vi "Update.vi"(8 "error in (no error)":errorcluster, 9 "Process Variable":dbl, 10 "Setpoint":dbl, 11 "PID in":refnum<class "PID.lvclass">) -> (0 "error out":errorcluster, 3 "PID out":refnum<class "PID.lvclass">)   [LabVIEW 2024, in "PID.lvlib" / "PID.lvclass"]
uses:
  PID.lvclass
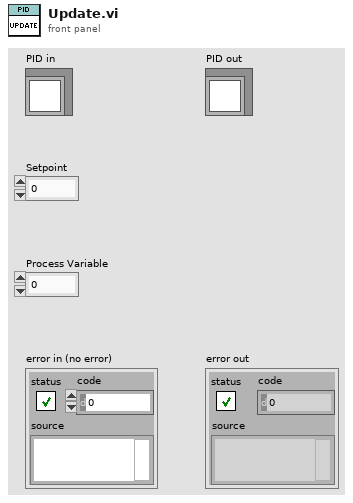
[diagram p1: front panel]
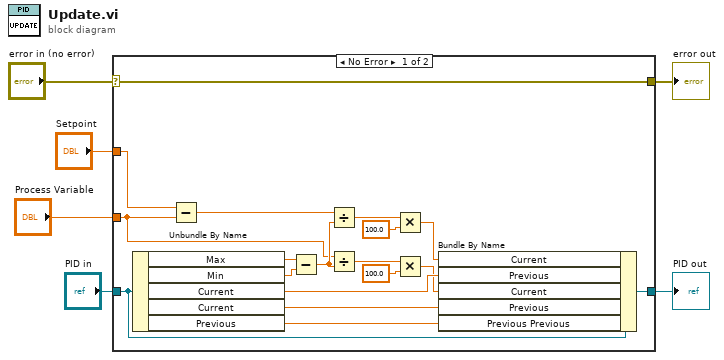
[diagram p0: block diagram]
diagram:
  n1 = case shown="No Error" "error in (no error)" {
    selector: "error in (no error)" -> [w24 w26]
    tunnel: [w24 w26] -> w5
    tunnel: [w14 w25] -> w3
    tunnel: "PID in" -> [w23 w25]
    tunnel: "Setpoint" -> [w22 _]
    tunnel: "Process Variable" -> [w10 _]
    frame No Error {
      n2 = Unbundle By Name(w23) -> ("Max"=w20:dbl, "Min"=w19:dbl, "Current"=w15:dbl, "Current"=w13:dbl, "Previous"=w12:dbl)
      n3 = Subtract(x=w22, y=w10) -> (x-y=w21:dbl)
      n4 = Subtract(x=w20, y=w19) -> (x-y=w11:dbl)
      n5 = Divide(x=w21, y=w11) -> (x/y=w18:dbl)
      n6 = Divide(x=w10, y=w11) -> (x/y=w9:dbl)
      n7 = Multiply(x=w18, y=100.0) -> (x*y=w16:dbl)
      n8 = Multiply(x=w9, y=100.0) -> (x*y=w7:dbl)
      n9 = Bundle By Name(cluster=w23, "Current"=w16, "Previous"=w15, "Current"=w7, "Previous"=w13, "Previous Previous"=w12) -> (w14:refnum<class "PID.lvclass">)
    }
    frame Error {
    }
  }
  "error out" <- w5
  "PID out" <- w3
